vi "ConfigureTrigger.vi"(8 "error in (no error)":errorcluster, 11 "Keysight44xx in":refnum<class "Keysight44xx.lvclass">) -> (0 "error out":errorcluster, 3 "Keysight44xx out":refnum<class "Keysight44xx.lvclass">)   [LabVIEW 2018, in "SpecAnPlugins.lvlib" / "Keysight44xx.lvclass"]
doc: "This function allows the user to configuree the Spectrum Analyser to acquire measurements based on a software, external, video or etc signal and the associated paramater such as level and slope."
uses:
  Keysight44xx.lvclass
  C:/Users/ico/Documents/Projects/NistPluggableModules/SpecAn/SpecAnPlugins/SpecAnBaseClass/SpecAnBase.lvclass
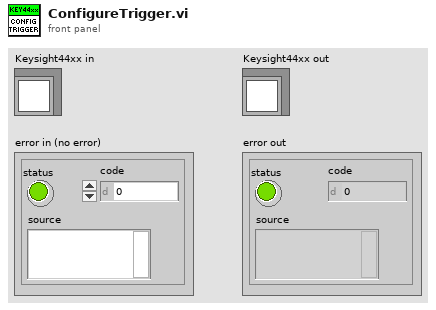
[diagram p1: front panel]
types:
  T1 = typedef "SpecAnPlugins.lvlib/SpecAnBase.lvclass/Acquisition.ctl" = cluster{"Handle":string, "Connected":bool, "Enabled":bool, "SweepModeContinuous":bool, "NumberOfSweeps":i32, "DetectorTypeAuto":bool, "DetectorType":i32, "VerticalScale":i32, "MaximumTime(seconds)":dbl}
  T2 = typedef "SpecAnPlugins.lvlib/SpecAnBase.lvclass/Trigger.ctl" = cluster{"TriggerLevel":dbl, "TriggerSlope":i32, "Trigger Source":i32}
  T3 = typedef "SpecAnPlugins.lvlib/Keysight44xx.lvclass/RFBurst.ctl" = cluster{"Frequency Selectivity (OFF)":bool, "Trigger Level Type (Absolute)":i32, "Narrow Pulse Discriminator (OFF)":bool}
  T4 = typedef "SpecAnPlugins.lvlib/Keysight44xx.lvclass/TV.ctl" = cluster{"Monitor Enabled (OFF)":bool, "SynchronizeSweep":bool, "SynchronizationLineNumber":i32, "TV Field (Any Field)":i32, "TV Signal Format (NTSC-M)":i32, "Trigger Source (Spectrum Analyzer)":i32}
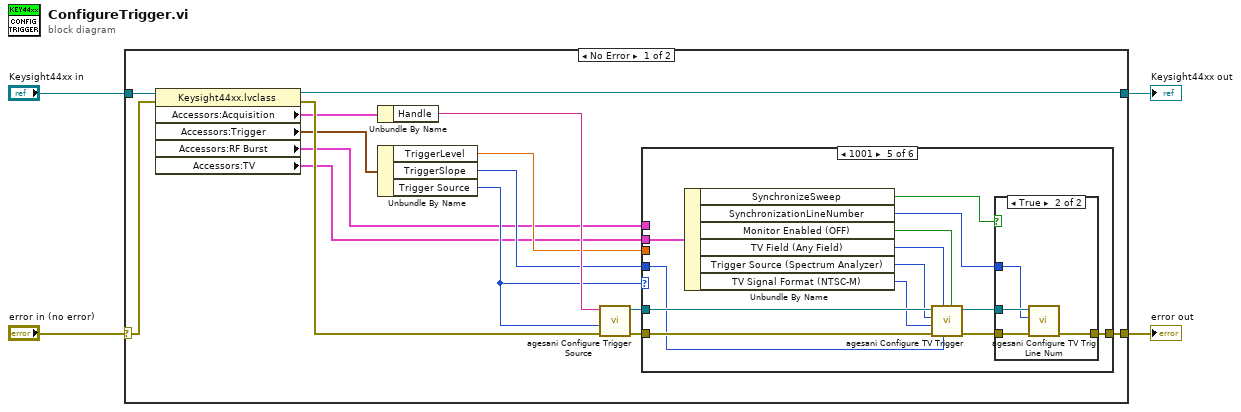
[diagram p0: block diagram]
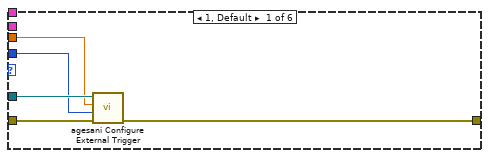
[diagram p2: hidden frame]
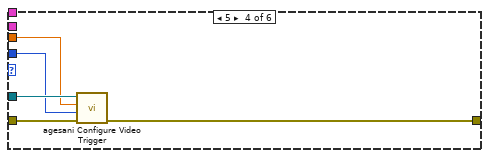
[diagram p5: hidden frame]
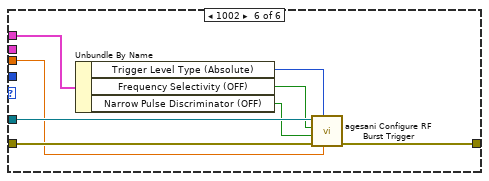
[diagram p7: hidden frame]
diagram:
  n1 = case shown="No Error" "error in (no error)" {
    selector: "error in (no error)" -> [w17 w58]
    tunnel: "Keysight44xx in" -> [w19 w59]
    tunnel: [w18 w59] -> w3
    tunnel: [w11 w58] -> w1
    frame No Error {
      n2 = property class="Keysight44xx.lvclass"(reference=w19, error in=w17) -> (reference out=w18:refnum<class "Keysight44xx.lvclass">, error out=w16:errorcluster, "Accessors:Acquisition"=w15:T1, "Accessors:Trigger"=w14:T2, "Accessors:RF Burst"=w6:T3, "Accessors:TV"=w5:T4)
      n3 = Unbundle By Name(w15) -> ("Handle"=w13:string)
      n4 = Unbundle By Name(w14) -> ("TriggerLevel"=w9:dbl, "TriggerSlope"=w8:i32, "Trigger Source"=w7:i32)
      n5 = call <instrlib>:"agesani Configure Trigger Source.vi"("error in (no error)"=w16, "trigger source (Immediate)"=w7, "instrument handle"=w13) -> ("error out"=w12:errorcluster, "instrument handle out"=w10:refnum<k15>)  [unwired: 7 in]
      n6 = case shown="1001" w7 {
        tunnel: w12 -> [w24 w25 w26 w31 w44 w57]
        tunnel: [w23 w25 w26 w30 w40 w56] -> w11
        tunnel: w10 -> [w22 _ _ w29 w43 w55]
        tunnel: w9 -> [w21 _ _ w28 _ w54]
        tunnel: w8 -> [w20 _ _ w27 w42 _]
        tunnel: w6 -> [_ _ _ _ _ w53]
        tunnel: w5 -> [_ _ _ _ w38 _]
        frame 1, Default {
          n7 = call <instrlib>:"agesani Configure External Trigger.vi"("error in (no error)"=w24, "external trigger polarity (Positive)"=w20, "external trigger level (1.5)"=w21, "instrument handle"=w22) -> ("error out"=w23:errorcluster)  [unwired: 6 in, 1 out]
        }
        frame 2 {
        }
        frame 4 {
        }
        frame 5 {
          n8 = call <instrlib>:"agesani Configure Video Trigger.vi"("error in (no error)"=w31, "video trigger slope (Positive)"=w27, "video trigger level (0.0)"=w28, "instrument handle"=w29) -> ("error out"=w30:errorcluster)  [unwired: 6 in, 1 out]
        }
        frame 1001 {
          n9 = Unbundle By Name(w38) -> ("SynchronizeSweep"=w37:bool, "SynchronizationLineNumber"=w36:i32, "Monitor Enabled (OFF)"=w35:bool, "TV Field (Any Field)"=w34:i32, "Trigger Source (Spectrum Analyzer)"=w32:i32, "TV Signal Format (NTSC-M)"=w33:i32)
          n10 = call <instrlib>:"agesani Configure TV Trigger.vi"("Monitor Enabled (Off)"=w35, "Trigger Polarity (Positive)"=w42, "TV Field (Any Field)"=w34, "error in (no error)"=w44, "TV Signal Format (NTSC-M)"=w33, "Trigger Source (Spectrum Analyzer)"=w32, "instrument handle"=w43) -> ("error out"=w41:errorcluster, "instrument handle out"=w39:refnum<k15>)  [unwired: 3 in]
          n11 = case shown="True" w37 {
            tunnel: w41 -> [w45 w49]
            tunnel: [w45 w48] -> w40
            tunnel: w39 -> [_ w47]
            tunnel: w36 -> [_ w46]
            frame False {
            }
            frame True {
              n12 = call <instrlib>:"agesani Configure TV Trig Line Num.vi"("error in (no error)"=w49, "Line number (17)"=w46, "instrument handle"=w47) -> ("error out"=w48:errorcluster)  [unwired: 7 in, 1 out]
            }
          }
        }
        frame 1002 {
          n13 = Unbundle By Name(w53) -> ("Trigger Level Type (Absolute)"=w52:i32, "Frequency Selectivity (OFF)"=w51:bool, "Narrow Pulse Discriminator (OFF)"=w50:bool)
          n14 = call <instrlib>:"agesani Configure RF Burst Trigger.vi"("Trigger Level (-6.0)"=w54, "Trigger Level Type (Absolute)"=w52, "error in (no error)"=w57, "Narrow Pulse Discriminator (Off)"=w50, "Frequency Selectivity (Off)"=w51, "instrument handle"=w55) -> ("error out"=w56:errorcluster)  [unwired: 4 in, 1 out]
        }
      }
    }
    frame Error {
    }
  }
  "error out" <- w1
  "Keysight44xx out" <- w3
